vi "ADCP_Init_Session.vi"(8 "error in (no error)":errorcluster, 10 "ADCP Session Parameters":T1, 11 "ADCP in":refnum<class "ADCP.lvclass">) -> (0 "error out":errorcluster, 3 "ADCP out":refnum<class "ADCP.lvclass">)   [LabVIEW 2017, in "ADCP.lvclass"]
uses:
  ADCP.lvclass
  <vilib>/Instr/_visa.llb/VISA Flush IO Buffer Mask.ctl
  ADCP.lvclass/ADCP.ctl
  <vilib>/Instr/_visa.llb/VISA Configure Serial Port (Instr).vi
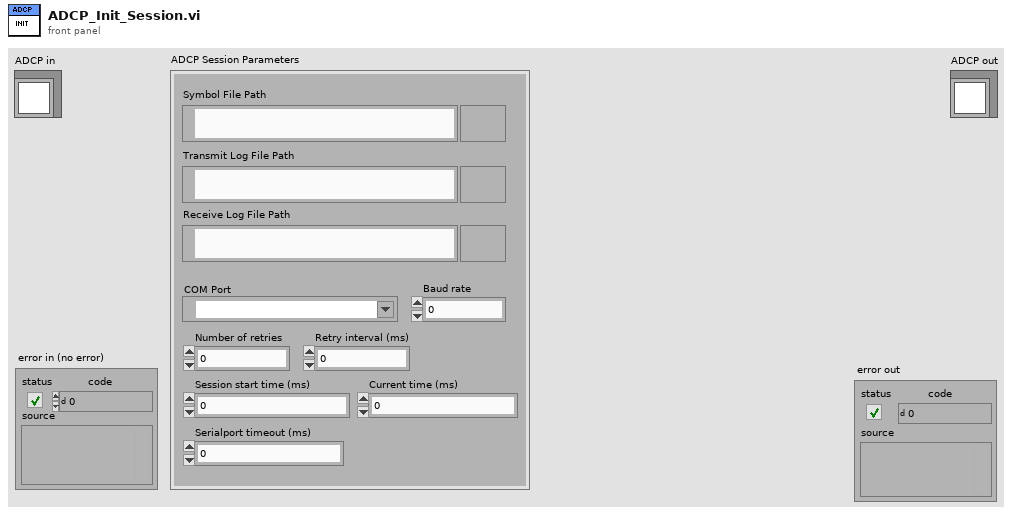
[diagram p1: front panel]
types:
  T1 = cluster{"Symbol File Path":path, "Transmit Log File Path":path, "Receive Log File Path":path, "COM Port":refnum<visa-resource-name>, "Baud rate":u32, "Number of retries":u16, "Retry interval (ms)":u16, "Session start time (ms)":u32, "Current time (ms)":u32, "Serialport timeout (ms)":u32}
  T2 = typedef "VISA Flush IO Buffer Mask.ctl" = u16
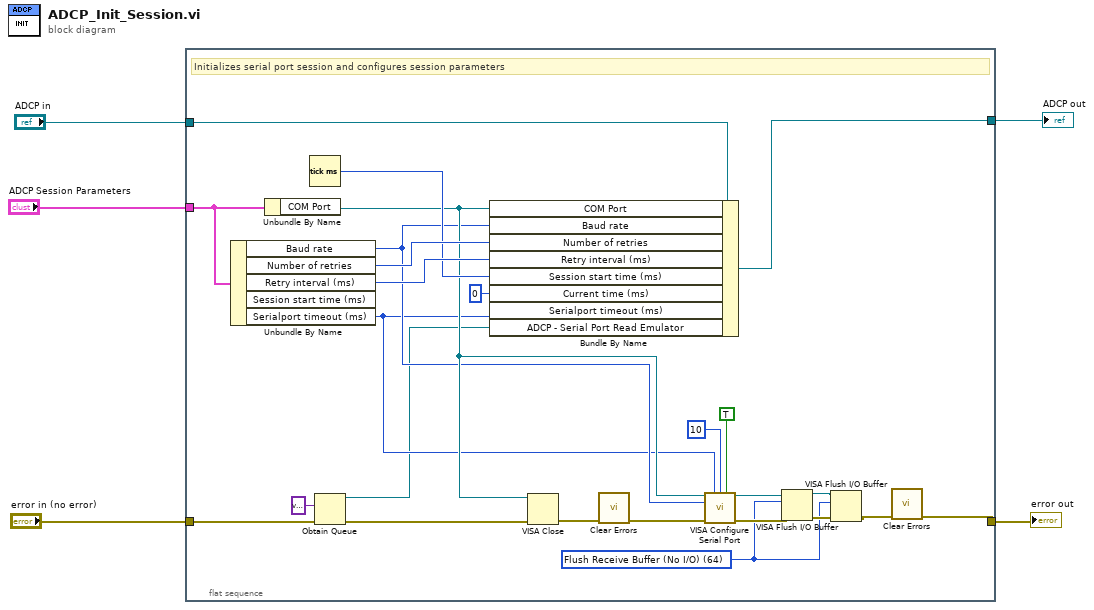
[diagram p0: block diagram]
diagram:
  n1 = flat-sequence {
    tunnel: "ADCP in" -> [w30]
    tunnel: [w29] -> w4
    tunnel: "ADCP Session Parameters" -> [w28]
    tunnel: "error in (no error)" -> [w11]
    tunnel: [w6] -> w2
    frame #0 {
      w13 = T2 64 items=["Flush Receive Buffer"=16, "Write Transmit Buffer to Device"=32, "Flush Receive Buffer (No I/O)"=64, "Flush Transmit Buffer"=128] ("Mask")
      # "Initializes serial port session and configures session parameters"
      n2 = Unbundle By Name(w28) -> ("Baud rate"=w18:u32, "Number of retries"=w27:u16, "Retry interval (ms)"=w26:u16, "Serialport timeout (ms)"=w12:u32)  [unwired: 1 out]
      n3 = Unbundle By Name(w28) -> ("COM Port"=w21:refnum<visa-resource-name>)
      n4 = Tick Count (ms)() -> (millisecond timer value=w25:u32)
      n5 = Obtain Queue(element data type=variant, error in (no error)=w11) -> (queue out=w9:refnum<queue>, error out=w10:errorcluster)  [unwired: 3 in, 1 out]
      n6 = Bundle By Name(cluster=w30, "COM Port"=w21, "Baud rate"=w18, "Number of retries"=w27, "Retry interval (ms)"=w26, "Session start time (ms)"=w25, "Current time (ms)"=u32 0 ("Session Parameters.Current time (ms)"), "Serialport timeout (ms)"=w12, "ADCP - Serial Port Read Emulator"=w9) -> (w29:refnum<class "ADCP.lvclass">)
      n7 = VISA Close(VISA resource name=w21, error in (no error)=w10) -> (error out=w23:errorcluster)
      n8 = call <vilib>:"Clear Errors.vi"("error in (no error)"=w23) -> ("error out"=w22:errorcluster)  [unwired: 5 in, 1 out]
      n9 = call-poly "VISA Configure Serial Port"("VISA resource name"=w21, "timeout (10sec)"=w12, "termination char\n(0xA = '\\n' = LF)"=u8 10 ("termination char\n(0xA = '\\n' = LF)"), "Enable Termination\nChar (T)"=TRUE ("Enable Termination\nChar (T)"), "baud rate (9600)"=w18, "error in (no error)"=w22) -> ("VISA resource name out"=w17:refnum<visa-resource-name>, "error out"=w16:errorcluster)  [unwired: 8 in]
      n10 = VISA Flush I/O Buffer(VISA resource name=w17, mask (16)=w13, error in (no error)=w16) -> (VISA resource name out=w15:refnum<visa-resource-name>, error out=w14:errorcluster)
      n11 = VISA Flush I/O Buffer(VISA resource name=w15, mask (16)=w13, error in (no error)=w14) -> (error out=w7:errorcluster)  [unwired: 1 out]
      n12 = call <vilib>:"Clear Errors.vi"("error in (no error)"=w7) -> ("error out"=w6:errorcluster)  [unwired: 5 in, 1 out]
    }
  }
  "ADCP out" <- w4
  "error out" <- w2
